vi "PH_PowerUnit_BaseClass.ProcCases.vi"(0 "i ref in":refnum<vi>, 1 "selector":string, 2 "Data":T1, 3 "call cluster":T2={"Object"="", "Selector"="", "CallType"=enum."synchronous", "Async Object"="", "Async Selector"="", "Data Descriptor"="", "Data"=[], "Error #"=0, "Expire"=0}, 5 "error in (no error)":errorcluster) -> (14 "i ref out":refnum<vi>, 17 "answer cluster":T2={"Object"="", "Selector"="", "CallType"=enum."synchronous", "Async Object"="", "Async Selector"="", "Data Descriptor"="", "Data"=[], "Error #"=0, "Expire"=0}, 19 "error out":errorcluster)   [LabVIEW 2014, in "PH_PowerUnit_BaseClass.lvlib"]
doc: "This method is called by a process from within the default case in the event loop. The methods of a class that are linked to events will be called from THIS method. Add your code here."
uses:
  PH_PowerUnit_BaseClass.lvlib
  CS_Core/CSSystem/CoreDefs/CoreDefs.call_type.ctl
  CS_Core/BaseProcess/BaseProcess.descriptor string definition.ctl
  CS_Core/CSSystem/CoreDefs/CoreDefs.rawDataType.ctl
  CS_Core/CSSystem/CoreLib/CoreLib.string 2 byte array.vi
  CS_Core/CSSystem/CoreLib/CoreLib.byte array 2 double.vi
  CS_Core/CSSystem/CoreLib/CoreLib.byte array 2 short.vi
  CS_Core/BaseProcess/BaseProcess.lvlib
  CS_Core/CSSystem/CoreLib/CoreLib.lvlib
  PH_Common/PH_Common.lvlib
  CS_Core/CAEObj/CAEObj.lvlib
  PH_StatusHandler/PH_StatusHandler.lvlib
  PH_PSDBWriter/PH_PSDBWriter.lvlib
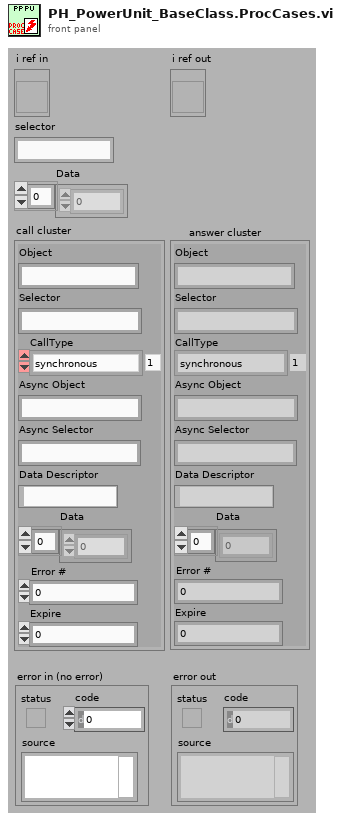
[diagram p1: front panel]
types:
  T1 = typedef "CoreDefs.rawDataType.ctl" = i8[]
  T2 = typedef "CoreDefs.call_type.ctl" = cluster{"Object":string, "Selector":string, "CallType":enum16{"simple", "synchronous", "asynchronous"}, "Async Object":string, "Async Selector":string, "Data Descriptor":T3, "Data":T1, "Error #":i32, "Expire":u32}
  T3 = typedef "BaseProcess.lvlib/BaseProcess.descriptor string definition.ctl" = string
  T4 = typedef "PH_PowerUnit_BaseClass.lvlib/PH_PowerUnit_BaseClass.i attribute.ctl" = cluster{"Constructor finished":bool, "PU":cluster{"In use":bool, "Service ID in use":i32, "GUI Ref":refnum<vi>}, "Enabling":cluster{"State":T5, "GUI Ref":refnum<vi>}, "Timing":cluster{"Last Shot":dbl, "Time between Shots [Sec]":dbl, "Waiting Time over?":bool, "Service ID Waiting Time":i32, "GUI Ref":refnum<vi>, "Instance":cluster{"Status":T6, "linked?":bool, "GUI Ref":refnum<vi>}}, "Sequencer":cluster{"SM State":string, "GUI Ref":refnum<vi>, "linked":bool}, "Subscribed Trendmssgs":cluster{"Tagname":string, "Status":T6, "linked?":bool, "Shot Condition":T6, "GUI Ref":refnum<vi>}[], "PP PU":T7, "Default Voltage (V)":dbl, "GUI Refs":T8, "PSDB data":cluster{"Shot Voltage [V]":dbl, "State TO SM":T9, "Write 2 early":bool}, "State TO SM":T9}
  T5 = typedef "PH_SystemInformation.lvlib/PH_SystemInformationEnabling State.ctl" = i32
  T6 = typedef "PH_StatusHandler.lvlib/PH_StatusHandler.Status.ctl" = i16
  T7 = typedef "PH_PP_Common.lvlib/PH_PP_Common.PUs.ctl" = enum16{"no Info", "PA-19mm-1", "PA-19mm-2", "PA-45mm-PILC", "PA-45mm-MAIN", "MA-PU-1", "MA-PU-2", "MA-PU-3", "MA-PU-4", "MA-PU-5", "MA-PU-6", "MA-FR", "MA-PILC", "PA-45mm-DP"}
  T8 = typedef "PH_PowerUnit_BaseClass.lvlib/PH_PowerUnit_BaseClass.GUI Refs.ctl" = cluster{"Delete Inst":refnum<vi>, "State TO SM":refnum<vi>, "State SM":refnum<vi>, "Fire":refnum<vi>}
  T9 = typedef "PH_PowerUnit_BaseClass.lvlib/PH_PowerUnit_BaseClass.SM States.ctl" = enum16{".", "Stand by", "Switch PU on", "Configure", "Set Default Voltage", "Set STANDBY", "Set READY", "Wait for Shot Cmd", "Open Dump Rods", "Open Ross Relais", "Close Ross Relais", "Switch PSU on", "Switch PSU off", "Charge", "Switch GD Channel on", "Close Dump Rods", "Rods-TO", "RR-TO", "PSU-TO", "Trigger-TO"}
  T10 = typedef "PH_PSDBWriter.lvlib/PH_PSDBWriter.PHELIX-Subsystems.ctl" = i32
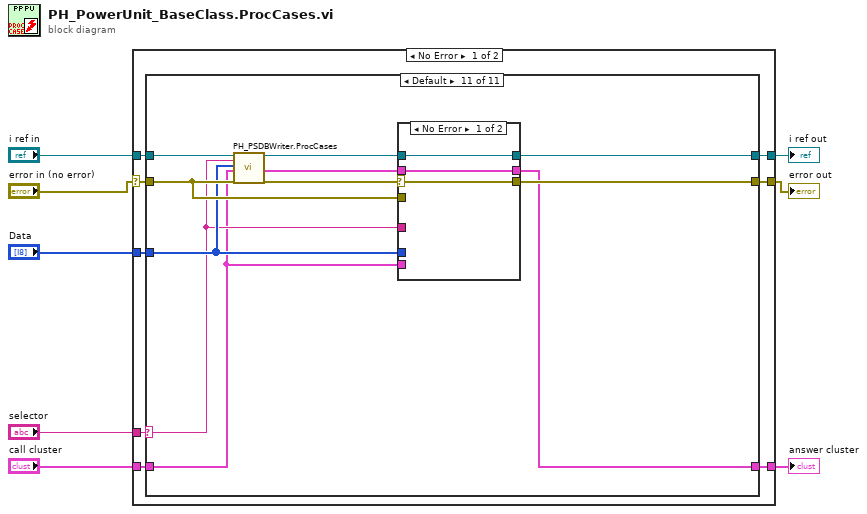
[diagram p0: block diagram]
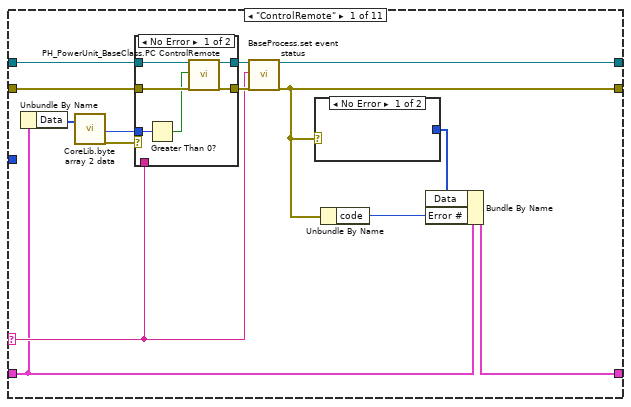
[diagram p2: hidden frame]
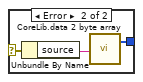
[diagram p3: hidden frame]
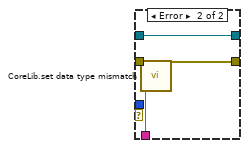
[diagram p4: hidden frame]
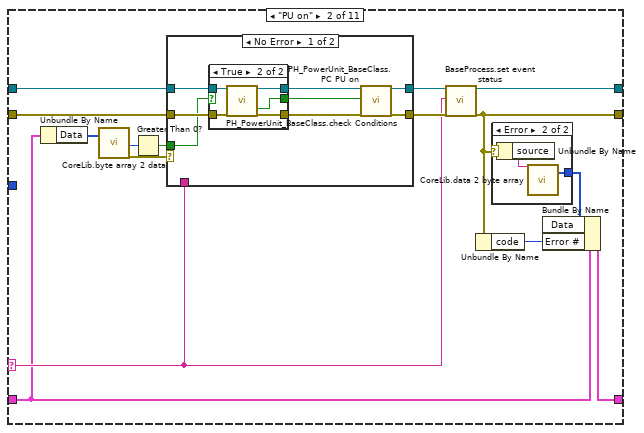
[diagram p5: hidden frame]
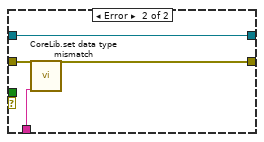
[diagram p8: hidden frame]
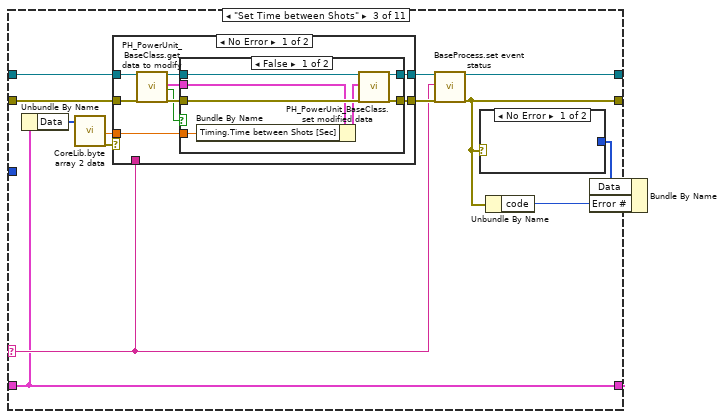
[diagram p9: hidden frame]
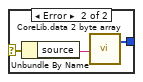
[diagram p10: hidden frame]
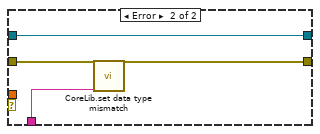
[diagram p12: hidden frame]
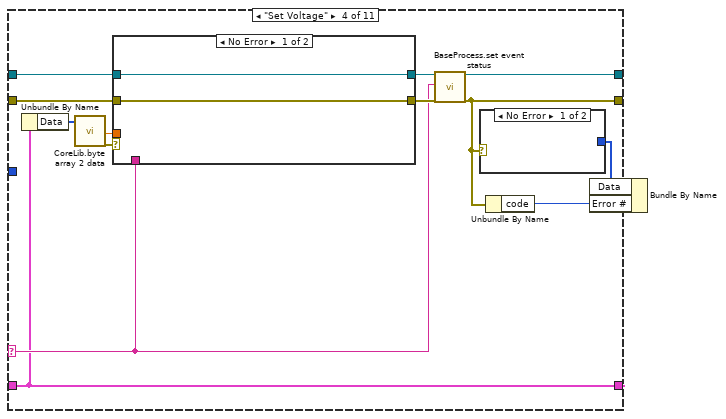
[diagram p13: hidden frame]
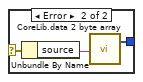
[diagram p14: hidden frame]
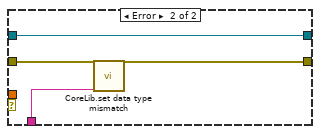
[diagram p15: hidden frame]
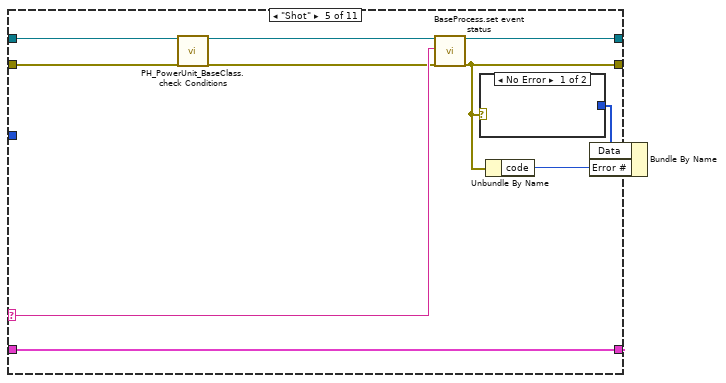
[diagram p16: hidden frame]
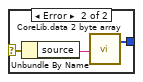
[diagram p17: hidden frame]
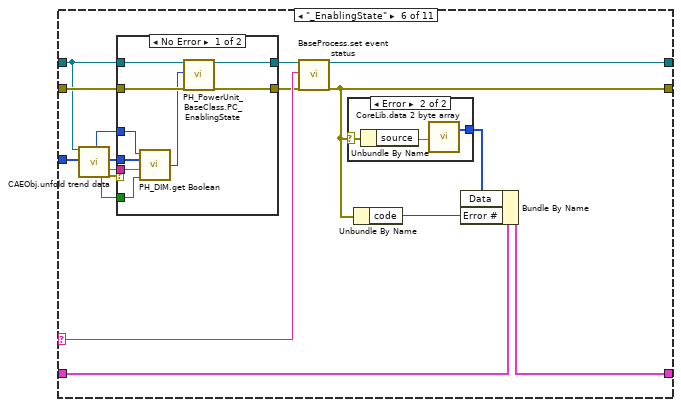
[diagram p18: hidden frame]
diagram:
  n1 = case shown="No Error" "error in (no error)" {
    selector: "error in (no error)" -> [w9 w345]
    tunnel: "selector" -> [w16 _]
    tunnel: [w15 w344] -> w7
    tunnel: "call cluster" -> [w14 w344]
    tunnel: "i ref in" -> [w13 w346]
    tunnel: [w12 w346] -> w4
    tunnel: [w11 w345] -> w3
    tunnel: "Data" -> [w10 _]
    frame No Error {
      n2 = case shown="Default" w16 {
        selector: w16 -> [w19 w50 w87 w126 w150 w162 w191 w221 w256 w290 w323]
        tunnel: w13 -> [w30 w58 w95 w134 w147 w172 w202 w232 w254 w283 w332]
        tunnel: [w21 w52 w89 w128 w152 w163 w193 w223 w260 w294 w329] -> w12
        tunnel: w14 -> [w18 w49 w86 w125 w149 w161 w190 w220 w258 w292 w322]
        tunnel: [w17 w48 w85 w124 w148 w160 w189 w219 w257 w291 w325] -> w15
        tunnel: w9 -> [w29 w57 w94 w133 w145 w174 w204 w234 w265 w282 w327]
        tunnel: [w20 w51 w88 w127 w151 w164 w192 w222 w259 w293 w331] -> w11
        tunnel: w10 -> [_ _ _ _ _ w173 w203 w233 w255 w284 w324]
        frame "ControlRemote" {
          n3 = Unbundle By Name(w18) -> ("Data"=w28:T1)
          n4 = call-poly "CoreLib.byte array 2 data.vi"("byteArray"=w28) -> ("i16"=w26:i16, "error out"=w27:errorcluster)  [unwired: 16 in, 1 out]
          n5 = case shown="No Error" w27 {
            tunnel: [w35 w43] -> w22
            tunnel: w30 -> [w39 w43]
            tunnel: w29 -> [w38 w42]
            tunnel: [w34 w41] -> w23
            tunnel: w19 -> [_ w40]
            tunnel: w26 -> [w37 _]
            frame No Error {
              n6 = Greater Than 0?(x=w37) -> (x > 0?=w36:bool)
              n7 = call "PH_PowerUnit_BaseClass.PC ControlRemote.vi"("i ref in"=w39, "Remote controlled?"=w36, "error in (no error)"=w38) -> ("i ref out"=w35:refnum<vi>, "error out"=w34:errorcluster)  [unwired: 15 in]
            }
            frame Error {
              n8 = call "CoreLib.set data type mismatch.vi"("error in (no error)"=w42, "error source"=w40) -> ("error out"=w41:errorcluster)  [unwired: 17 in]
            }
          }
          n9 = call "BaseProcess.set event status.vi"("i ref in"=w22, "EventStatus"=w19, "error in (no error)"=w23) -> ("i ref out"=w21:refnum<vi>, "error out"=w20:errorcluster)  [unwired: 14 in, 1 out]
          n10 = case shown="No Error" w20 {
            selector: w20 -> [_ w33]
            tunnel: [_ w31] -> w24
            frame No Error {
            }
            frame Error {
              n11 = Unbundle By Name(w33) -> ("source"=w32:string)
              n12 = call-poly "CoreLib.data 2 byte array.vi"("string"=w32) -> ("byteArray out"=w31:T1)  [unwired: 18 in]
            }
          }
          n13 = Unbundle By Name(w20) -> ("code"=w25:i32)
          n14 = Bundle By Name(cluster=w18, "Data"=w24, "Error #"=w25) -> (w17:T2)
        }
        frame "PU on" {
          n15 = Unbundle By Name(w49) -> ("Data"=w47:T1)
          n16 = call-poly "CoreLib.byte array 2 data.vi"("byteArray"=w47) -> ("i16"=w46:i16, "error out"=w44:errorcluster)  [unwired: 16 in, 1 out]
          n17 = Greater Than 0?(x=w46) -> (x > 0?=w45:bool)
          n18 = case shown="No Error" w44 {
            tunnel: w58 -> [w65 w79]
            tunnel: [w68 w79] -> w53
            tunnel: w57 -> [w69 w81]
            tunnel: [w67 w80] -> w54
            tunnel: w50 -> [_ w78]
            tunnel: w45 -> [w63 _]
            frame No Error {
              n19 = case shown="True" w63 {
                selector: w63 -> [w70 _]
                tunnel: w69 -> [w71 w77]
                tunnel: [w71 w76] -> w66
                tunnel: w65 -> [w72 w75]
                tunnel: [w72 w74] -> w64
                tunnel: [w70 w73] -> w62
                frame False {
                }
                frame True {
                  n20 = call "PH_PowerUnit_BaseClass.check Conditions.vi"("VI in"=w75, "error in (no error)"=w77) -> ("VI out"=w74:refnum<vi>, "Ready to switch PU on"=w73:bool, "error out"=w76:errorcluster)  [unwired: 14 in, 1 out]
                }
              }
              n21 = call "PH_PowerUnit_BaseClass.PC PU on.vi"("i ref in"=w64, "PU on"=w62, "error in (no error)"=w66) -> ("i ref out"=w68:refnum<vi>, "error out"=w67:errorcluster)  [unwired: 15 in]
            }
            frame Error {
              n22 = call "CoreLib.set data type mismatch.vi"("error in (no error)"=w81, "error source"=w78) -> ("error out"=w80:errorcluster)  [unwired: 17 in]
            }
          }
          n23 = call "BaseProcess.set event status.vi"("i ref in"=w53, "EventStatus"=w50, "error in (no error)"=w54) -> ("i ref out"=w52:refnum<vi>, "error out"=w51:errorcluster)  [unwired: 14 in, 1 out]
          n24 = Unbundle By Name(w51) -> ("code"=w56:i32)
          n25 = case shown="Error" w51 {
            selector: w51 -> [_ w61]
            tunnel: [_ w59] -> w55
            frame No Error {
            }
            frame Error {
              n26 = Unbundle By Name(w61) -> ("source"=w60:string)
              n27 = call-poly "CoreLib.data 2 byte array.vi"("string"=w60) -> ("byteArray out"=w59:T1)  [unwired: 18 in]
            }
          }
          n28 = Bundle By Name(cluster=w49, "Data"=w55, "Error #"=w56) -> (w48:T2)
        }
        frame "Set Time between Shots" {
          n29 = Unbundle By Name(w86) -> ("Data"=w84:T1)
          n30 = call-poly "CoreLib.byte array 2 data.vi"("byteArray"=w84) -> ("d64"=w82:dbl, "error out"=w83:errorcluster)  [unwired: 16 in, 1 out]
          n31 = case shown="No Error" w83 {
            tunnel: [w103 w120] -> w90
            tunnel: w95 -> [w107 w120]
            tunnel: w94 -> [w99 w119]
            tunnel: [w104 w118] -> w91
            tunnel: w87 -> [_ w117]
            tunnel: w82 -> [w101 _]
            frame No Error {
              n32 = call "PH_PowerUnit_BaseClass.get data to modify.vi"("i ref in"=w107, "error in (no error)"=w99) -> ("i ref out"=w106:refnum<vi>, "i attribute"=w102:T4, "timed out"=w100:bool, "error out"=w105:errorcluster)  [unwired: 14 in]
              n33 = case shown="False" w100 {
                tunnel: w106 -> [w114 w116]
                tunnel: w105 -> [w113 w115]
                tunnel: [w112 w115] -> w104
                tunnel: [w111 w116] -> w103
                tunnel: w102 -> [w110 _]
                tunnel: w101 -> [w108 _]
                frame False {
                  n34 = Bundle By Name(cluster=w110, "Timing.Time between Shots [Sec]"=w108) -> (w109:T4)
                  n35 = call "PH_PowerUnit_BaseClass.set modified data.vi"("i ref in"=w114, "i attribute"=w109, "error in (no error)"=w113) -> ("i ref out"=w111:refnum<vi>, "error out"=w112:errorcluster)  [unwired: 15 in]
                }
                frame True {
                }
              }
            }
            frame Error {
              n36 = call "CoreLib.set data type mismatch.vi"("error in (no error)"=w119, "error source"=w117) -> ("error out"=w118:errorcluster)  [unwired: 17 in]
            }
          }
          n37 = call "BaseProcess.set event status.vi"("i ref in"=w90, "EventStatus"=w87, "error in (no error)"=w91) -> ("i ref out"=w89:refnum<vi>, "error out"=w88:errorcluster)  [unwired: 14 in, 1 out]
          n38 = case shown="No Error" w88 {
            selector: w88 -> [_ w98]
            tunnel: [_ w96] -> w92
            frame No Error {
            }
            frame Error {
              n39 = Unbundle By Name(w98) -> ("source"=w97:string)
              n40 = call-poly "CoreLib.data 2 byte array.vi"("string"=w97) -> ("byteArray out"=w96:T1)  [unwired: 18 in]
            }
          }
          n41 = Unbundle By Name(w88) -> ("code"=w93:i32)
          n42 = Bundle By Name(cluster=w86, "Data"=w92, "Error #"=w93) -> (w85:T2)
        }
        frame "Set Voltage" {
          n43 = Unbundle By Name(w125) -> ("Data"=w123:T1)
          n44 = call-poly "CoreLib.byte array 2 data.vi"("byteArray"=w123) -> ("d64"=w121:dbl, "error out"=w122:errorcluster)  [unwired: 16 in, 1 out]
          n45 = case shown="No Error" w122 {
            tunnel: [w139 w143] -> w129
            tunnel: w134 -> [w139 w143]
            tunnel: w133 -> [w138 w142]
            tunnel: [w138 w141] -> w130
            tunnel: w126 -> [_ w140]
            tunnel: w121 -> [_ _]
            frame No Error {
            }
            frame Error {
              n46 = call "CoreLib.set data type mismatch.vi"("error in (no error)"=w142, "error source"=w140) -> ("error out"=w141:errorcluster)  [unwired: 17 in]
            }
          }
          n47 = call "BaseProcess.set event status.vi"("i ref in"=w129, "EventStatus"=w126, "error in (no error)"=w130) -> ("i ref out"=w128:refnum<vi>, "error out"=w127:errorcluster)  [unwired: 14 in, 1 out]
          n48 = case shown="No Error" w127 {
            selector: w127 -> [_ w137]
            tunnel: [_ w135] -> w131
            frame No Error {
            }
            frame Error {
              n49 = Unbundle By Name(w137) -> ("source"=w136:string)
              n50 = call-poly "CoreLib.data 2 byte array.vi"("string"=w136) -> ("byteArray out"=w135:T1)  [unwired: 18 in]
            }
          }
          n51 = Unbundle By Name(w127) -> ("code"=w132:i32)
          n52 = Bundle By Name(cluster=w125, "Data"=w131, "Error #"=w132) -> (w124:T2)
        }
        frame "Shot" {
          n53 = call "PH_PowerUnit_BaseClass.check Conditions.vi"("VI in"=w147, "error in (no error)"=w145) -> ("VI out"=w146:refnum<vi>, "error out"=w144:errorcluster)  [unwired: 14 in, 2 out]
          n54 = call "BaseProcess.set event status.vi"("i ref in"=w146, "EventStatus"=w150, "error in (no error)"=w144) -> ("i ref out"=w152:refnum<vi>, "error out"=w151:errorcluster)  [unwired: 14 in, 1 out]
          n55 = case shown="No Error" w151 {
            selector: w151 -> [_ w157]
            tunnel: [_ w155] -> w153
            frame No Error {
            }
            frame Error {
              n56 = Unbundle By Name(w157) -> ("source"=w156:string)
              n57 = call-poly "CoreLib.data 2 byte array.vi"("string"=w156) -> ("byteArray out"=w155:T1)  [unwired: 18 in]
            }
          }
          n58 = Unbundle By Name(w151) -> ("code"=w154:i32)
          n59 = Bundle By Name(cluster=w149, "Data"=w153, "Error #"=w154) -> (w148:T2)
        }
        frame "_EnablingState" {
          n60 = call "CAEObj.unfold trend data.vi"("i ref in"=w172, "raw trend data"=w173) -> ("quality"=w170:i32, "no link"=w168:bool, "data"=w167:i8[], "typeDescriptor"=w169:string, "error out"=w171:errorcluster)  [unwired: 9 in, 4 out]
          n61 = case shown="No Error" w171 {
            tunnel: [w179 w188] -> w158
            tunnel: w172 -> [w186 w188]
            tunnel: w174 -> [w185 w187]
            tunnel: [w178 w187] -> w159
            tunnel: w170 -> [w184 _]
            tunnel: w169 -> [w183 _]
            tunnel: w168 -> [w182 _]
            tunnel: w167 -> [w181 _]
            frame No Error {
              n62 = call "PH_DIM.get Boolean.vi"("no link"=w182, "typeDescriptor"=w183, "data"=w181, "quality"=w184) -> ("Value"=w180:i32)
              n63 = call "PH_PowerUnit_BaseClass.PC_EnablingState.vi"("i ref in"=w186, "Tagvalue"=w180, "error in (no error)"=w185) -> ("i ref out"=w179:refnum<vi>, "error out"=w178:errorcluster)  [unwired: 15 in]
            }
            frame Error {
            }
          }
          n64 = call "BaseProcess.set event status.vi"("i ref in"=w158, "EventStatus"=w162, "error in (no error)"=w159) -> ("i ref out"=w163:refnum<vi>, "error out"=w164:errorcluster)  [unwired: 14 in, 1 out]
          n65 = case shown="Error" w164 {
            selector: w164 -> [_ w177]
            tunnel: [_ w175] -> w165
            frame No Error {
            }
            frame Error {
              n66 = Unbundle By Name(w177) -> ("source"=w176:string)
              n67 = call-poly "CoreLib.data 2 byte array.vi"("string"=w176) -> ("byteArray out"=w175:T1)  [unwired: 18 in]
            }
          }
          n68 = Unbundle By Name(w164) -> ("code"=w166:i32)
          n69 = Bundle By Name(cluster=w161, "Data"=w165, "Error #"=w166) -> (w160:T2)
        }
        frame "TimingInstanceStatus" {
          n70 = call "CAEObj.unfold trend data.vi"("i ref in"=w202, "raw trend data"=w203) -> ("no link"=w198:bool, "data"=w199:i8[], "typeDescriptor"=w200:string, "error out"=w201:errorcluster)  [unwired: 9 in, 5 out]
          n71 = case shown="No Error" w201 {
            tunnel: [w209 w217] -> w194
            tunnel: w202 -> [w215 w217]
            tunnel: w204 -> [w214 w216]
            tunnel: [w208 w216] -> w195
            tunnel: w200 -> [w213 _]
            tunnel: w199 -> [w211 _]
            tunnel: w198 -> [w212 _]
            frame No Error {
              n72 = call "PH_StatusHandler.get Status DIM Service.vi"("no link"=w212, "typeDescriptor"=w213, "data"=w211) -> ("Status"=w210:T6)  [unwired: 1 in]
              n73 = call "PH_PowerUnit_BaseClass.PC_Timing Instance Status.vi"("i ref in"=w215, "Status"=w210, "not linked?"=w212, "error in (no error)"=w214) -> ("i ref out"=w209:refnum<vi>, "error out"=w208:errorcluster)  [unwired: 14 in]
            }
            frame Error {
            }
          }
          n74 = call "BaseProcess.set event status.vi"("i ref in"=w194, "EventStatus"=w191, "error in (no error)"=w195) -> ("i ref out"=w193:refnum<vi>, "error out"=w192:errorcluster)  [unwired: 14 in, 1 out]
          n75 = case shown="No Error" w192 {
            selector: w192 -> [_ w207]
            tunnel: [_ w205] -> w196
            frame No Error {
            }
            frame Error {
              n76 = Unbundle By Name(w207) -> ("source"=w206:string)
              n77 = call-poly "CoreLib.data 2 byte array.vi"("string"=w206) -> ("byteArray out"=w205:T1)  [unwired: 18 in]
            }
          }
          n78 = Unbundle By Name(w192) -> ("code"=w197:i32)
          n79 = Bundle By Name(cluster=w190, "Data"=w196, "Error #"=w197) -> (w189:T2)
        }
        frame "_Trendmssgs" {
          n80 = call "CAEObj.unfold trend data.vi"("i ref in"=w232, "raw trend data"=w233) -> ("no link"=w228:bool, "data"=w229:i8[], "serviceName"=w218:string, "typeDescriptor"=w230:string, "error out"=w231:errorcluster)  [unwired: 9 in, 4 out]
          n81 = case shown="No Error" w231 {
            tunnel: [w240 w248] -> w224
            tunnel: w232 -> [w246 w248]
            tunnel: w234 -> [w245 w247]
            tunnel: [w239 w247] -> w225
            tunnel: w230 -> [w244 _]
            tunnel: w229 -> [w242 _]
            tunnel: w228 -> [w243 _]
            tunnel: w218 -> [w238 _]
            frame No Error {
              n82 = call "PH_StatusHandler.get Status DIM Service.vi"("no link"=w243, "typeDescriptor"=w244, "data"=w242) -> ("Status"=w241:T6)  [unwired: 1 in]
              n83 = call "PH_PowerUnit_BaseClass.PC_TrendMssgs.vi"("i ref in"=w246, "Instance"=w238, "Status"=w241, "not linked?"=w243, "error in (no error)"=w245) -> ("i ref out"=w240:refnum<vi>, "error out"=w239:errorcluster)  [unwired: 13 in]
            }
            frame Error {
            }
          }
          n84 = call "BaseProcess.set event status.vi"("i ref in"=w224, "EventStatus"=w221, "error in (no error)"=w225) -> ("i ref out"=w223:refnum<vi>, "error out"=w222:errorcluster)  [unwired: 14 in, 1 out]
          n85 = case shown="No Error" w222 {
            selector: w222 -> [_ w237]
            tunnel: [_ w235] -> w226
            frame No Error {
            }
            frame Error {
              n86 = Unbundle By Name(w237) -> ("source"=w236:string)
              n87 = call-poly "CoreLib.data 2 byte array.vi"("string"=w236) -> ("byteArray out"=w235:T1)  [unwired: 18 in]
            }
          }
          n88 = Unbundle By Name(w222) -> ("code"=w227:i32)
          n89 = Bundle By Name(cluster=w220, "Data"=w226, "Error #"=w227) -> (w219:T2)
        }
        frame "_SMStateSequencer" {
          n90 = call "CAEObj.unfold trend data.vi"("i ref in"=w254, "raw trend data"=w255) -> ("quality"=w249:i32, "no link"=w250:bool, "data"=w252:i8[], "typeDescriptor"=w251:string, "error out"=w253:errorcluster)  [unwired: 9 in, 4 out]
          n91 = case shown="No Error" w253 {
            tunnel: w254 -> [w275 w279]
            tunnel: [w270 w279] -> w261
            tunnel: w265 -> [w274 w278]
            tunnel: [w269 w278] -> w262
            tunnel: w252 -> [w277 _]
            tunnel: w251 -> [w276 _]
            tunnel: w250 -> [w272 _]
            tunnel: w249 -> [w271 _]
            frame No Error {
              n92 = call "PH_DIM.get String.vi"("no link"=w272, "typeDescriptor"=w276, "data"=w277, "quality"=w271) -> ("Output String"=w273:string)
              n93 = call "PH_PowerUnit_BaseClass.PC Seq SM.vi"("i ref in"=w275, "SM State"=w273, "no link"=w272, "error in"=w274) -> ("i ref out"=w270:refnum<vi>, "error out"=w269:errorcluster)  [unwired: 14 in]
            }
            frame Error {
            }
          }
          n94 = call "BaseProcess.set event status.vi"("i ref in"=w261, "EventStatus"=w256, "error in (no error)"=w262) -> ("i ref out"=w260:refnum<vi>, "error out"=w259:errorcluster)  [unwired: 14 in, 1 out]
          n95 = case shown="Error" w259 {
            selector: w259 -> [_ w268]
            tunnel: [_ w266] -> w263
            frame No Error {
            }
            frame Error {
              n96 = Unbundle By Name(w268) -> ("source"=w267:string)
              n97 = call-poly "CoreLib.data 2 byte array.vi"("string"=w267) -> ("byteArray out"=w266:T1)  [unwired: 18 in]
            }
          }
          n98 = Unbundle By Name(w259) -> ("code"=w264:i32)
          n99 = Bundle By Name(cluster=w258, "Data"=w263, "Error #"=w264) -> (w257:T2)
        }
        frame "_set_PSDB_Data" {
          n100 = call "CAEObj.unfold trend data.vi"("i ref in"=w283, "raw trend data"=w284) -> ("quality"=w285:i32, "no link"=w288:bool, "data"=w286:i8[], "typeDescriptor"=w287:string, "error out"=w289:errorcluster)  [unwired: 9 in, 4 out]
          n101 = case shown="No Error" w289 {
            tunnel: w282 -> [w304 w318]
            tunnel: [w308 w317] -> w281
            tunnel: [w307 w318] -> w280
            tunnel: w283 -> [w306 w317]
            tunnel: w288 -> [w298 _]
            tunnel: w287 -> [w300 _]
            tunnel: w286 -> [w301 _]
            tunnel: w285 -> [w299 _]
            frame No Error {
              n102 = call "PH_PSDBWriter.get Subsystem DIM Service.vi"("no link"=w298, "typeDescriptor"=w300, "data"=w301, "quality"=w299) -> ("PHELIX Subsystems"=w297:T10)
              n103 = call "PH_PSDBWriter.check PSDB writing condition.vi"("i ref in"=w306, "wanted Subsystem"=w297, "error IO"=w304) -> ("i ref out"=w305:refnum<vi>, "write PSDB?"=w302:bool, "error out"=w303:errorcluster)  [unwired: 14 in]
              n104 = case shown="True" w302 {
                tunnel: w303 -> [w309 w311]
                tunnel: [w310 w315] -> w308
                tunnel: [w309 w316] -> w307
                tunnel: w305 -> [w310 w312]
                frame False {
                }
                frame True {
                  n105 = call "PH_PowerUnit_BaseClass.write PSDB.vi"("i ref in"=w312, "error IO"=w311) -> ("i ref out"=w313:refnum<vi>, "error out"=w314:errorcluster)  [unwired: 16 in]
                  n106 = call "PH_PSDBWriter.evt call write PSDB.vi"("i ref in"=w313, "error in (no error)"=w314) -> ("i ref out"=w315:refnum<vi>, "error out"=w316:errorcluster)  [unwired: 16 in]
                }
              }
            }
            frame Error {
            }
          }
          n107 = call "BaseProcess.set event status.vi"("i ref in"=w281, "EventStatus"=w290, "error in (no error)"=w280) -> ("i ref out"=w294:refnum<vi>, "error out"=w293:errorcluster)  [unwired: 14 in, 1 out]
          n108 = Unbundle By Name(w293) -> ("code"=w296:i32)
          n109 = case shown="Error" w293 {
            selector: w293 -> [_ w321]
            tunnel: [_ w319] -> w295
            frame No Error {
            }
            frame Error {
              n110 = Unbundle By Name(w321) -> ("source"=w320:string)
              n111 = call-poly "CoreLib.data 2 byte array.vi"("string"=w320) -> ("byteArray out"=w319:T1)  [unwired: 18 in]
            }
          }
          n112 = Bundle By Name(cluster=w292, "Data"=w295, "Error #"=w296) -> (w291:T2)
        }
        frame Default {
          n113 = call "PH_PSDBWriter.ProcCases.vi"("i ref in"=w332, "selector"=w323, "Data"=w324, "call cluster"=w322, "error in"=w327) -> ("i ref out"=w330:refnum<vi>, "answer cluster"=w326:T2, "error out"=w328:errorcluster)  [unwired: 12 in]
          n114 = case shown="No Error" w328 {
            selector: w328 -> [w335 _]
            tunnel: w327 -> [_ w343]
            tunnel: [w335 w342] -> w331
            tunnel: w330 -> [w334 w341]
            tunnel: [w334 w340] -> w329
            tunnel: w326 -> [w333 _]
            tunnel: [w333 w339] -> w325
            tunnel: w324 -> [_ w338]
            tunnel: w323 -> [_ w337]
            tunnel: w322 -> [_ w336]
            frame No Error {
            }
            frame Error {
              n115 = call "PH_StatusHandler.ProcCases.vi"("i ref in"=w341, "selector"=w337, "Data"=w338, "call cluster"=w336, "error in (no error)"=w343) -> ("i ref out"=w340:refnum<vi>, "answer cluster"=w339:T2, "error out"=w342:errorcluster)  [unwired: 12 in]
            }
          }
        }
      }
    }
    frame Error {
    }
  }
  "answer cluster" <- w7
  "i ref out" <- w4
  "error out" <- w3
